vi "Store Ref to Configuration.vi"(8 "error in (no error)":errorcluster, 10 "Control Name":string="Configuration", 11 "Measure Object in":refnum<class "Da Base.lvclass">) -> (0 "error out":errorcluster, 3 "Measure Object out":refnum<class "Da Base.lvclass">)   [LabVIEW 2016, in "Da Base.lvclass"]
uses:
  Da Base.lvclass
  Da Base.lvclass/Da Base.ctl
  Read Front Panel ref.vi
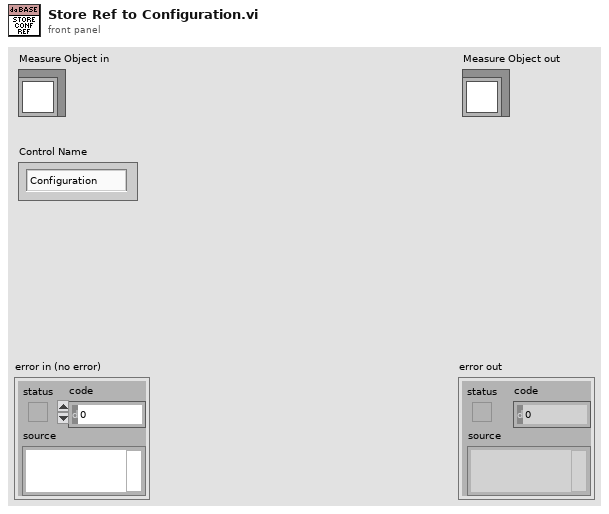
[diagram p1: front panel]
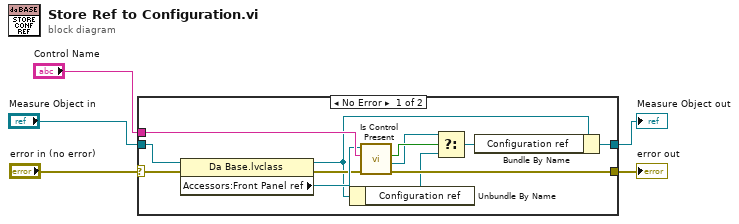
[diagram p0: block diagram]
diagram:
  n1 = case shown="No Error" "error in (no error)" {
    selector: "error in (no error)" -> [w10 w19]
    tunnel: [w9 w19] -> w4
    tunnel: [w8 w18] -> w2
    tunnel: "Measure Object in" -> [w14 w18]
    tunnel: "Control Name" -> [w17 _]
    frame No Error {
      n2 = property class="Da Base.lvclass"(reference=w14, error in=w10) -> (reference out=w7:refnum<class "Da Base.lvclass">, error out=w15:errorcluster, "Accessors:Front Panel ref"=w16:refnum<vi>)
      n3 = Unbundle By Name(w7) -> ("Configuration ref"=w6:refnum<vi>)
      n4 = call "Is Control Present.vi"("Error In"=w15, "Control label"=w17, "VI ref"=w16) -> ("Error Out"=w9:errorcluster, "Ctl Refnum"=w12:refnum<vi>, "Present"=w13:bool)  [unwired: 5 in, 1 out]
      n5 = Select(t=w12, s=w13, f=w6) -> (s? t:f=w11:refnum<vi>)
      n6 = Bundle By Name(cluster=w7, "Configuration ref"=w11) -> (w8:refnum<class "Da Base.lvclass">)
    }
    frame Error {
    }
  }
  "error out" <- w4
  "Measure Object out" <- w2
